vi "cwlaser.vi"() -> ()   [LabVIEW 2017]
panel:
  in  "power (mW)":dbl
  in  "wavelength":dbl format="%#_13g"
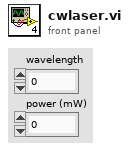
[diagram p1: front panel]
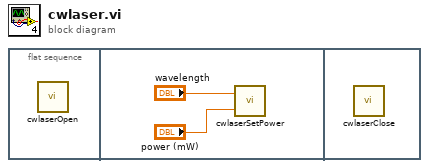
[diagram p0: block diagram]
diagram:
  n1 = flat-sequence {
    frame #0 {
      n2 = call "cwlaserOpen.vi"() -> ()  [unwired: 4 in]
    }
    frame #1 {
      n3 = call "cwlaserSetPower.vi"("power (mW)"="power (mW)", "wavelength"="wavelength") -> ()  [unwired: 1 in]
    }
    frame #2 {
      n4 = call "cwlaserClose.vi"() -> ()  [unwired: 3 in]
    }
  }
